vi "Wash Entry Display.vi"(0 "Wash Entry Text":string, 1 "Wash Entry Color":cluster{u32, u32}[](array[cluster])=[{4390733, 6618880}], 3 "error in (no error)":errorcluster, 4 "Wash Entry Reference":refnum<vi>) -> (10 "error out":errorcluster)   [LabVIEW 2020]
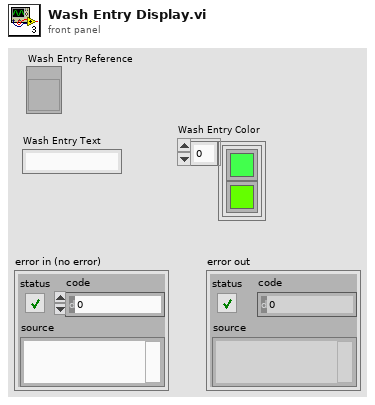
[diagram p1: front panel]
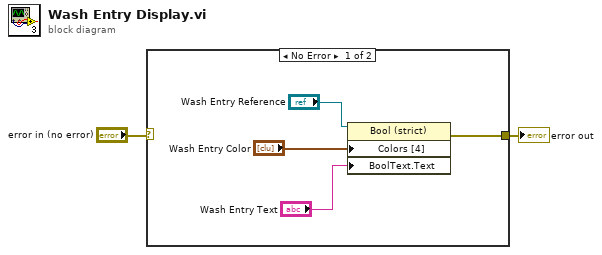
[diagram p0: block diagram]
diagram:
  n1 = case shown="No Error" "error in (no error)" {
    selector: "error in (no error)" -> [_ w7]
    tunnel: [w3 w7] -> w1
    frame No Error {
      n2 = property class="Bool (strict)"(reference="Wash Entry Reference", "Colors [4]"="Wash Entry Color", "BoolText.Text"="Wash Entry Text") -> (error out=w3:errorcluster)  [unwired: 1 in, 1 out]
    }
    frame Error {
    }
  }
  "error out" <- w1
